vi "C8855-01_ReadData.vi"(8 "MainD":T1 {"G_DIM" format="%.5f"}) -> (0 "MainDR":T1 {"G_DIM" format="%.5f"}, 1 "RR2":u8, 2 "RR1":u8, 3 "Error":bool)   [LabVIEW 2017]
uses:
  C8855_MainD.ctl
  C8855-01api.dll
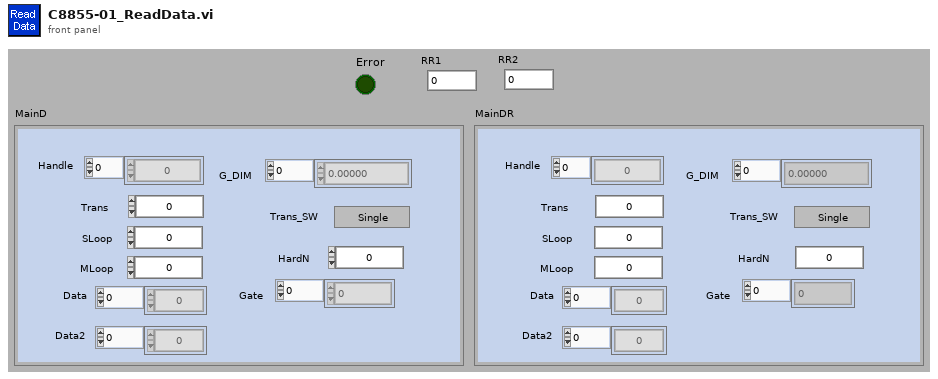
[diagram p1: front panel]
types:
  T1 = typedef "C8855_MainD.ctl" = cluster{"Handle":i64[], "G_DIM":dbl[], "Trans":u16, "Trans_SW":bool, "HardN":i32, "Gate":u8[], "Data":u32[], "Data2":u32[], "SLoop":i32, "MLoop":i32}
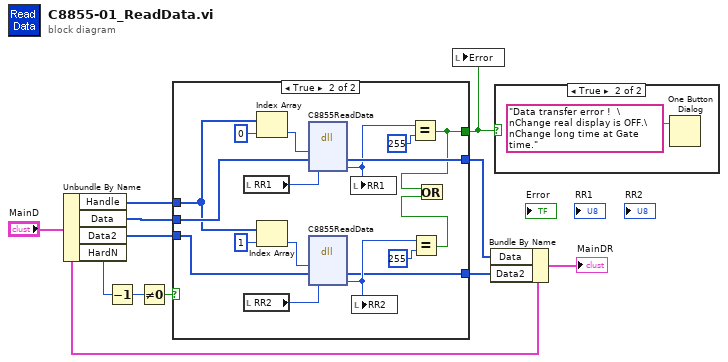
[diagram p0: block diagram]
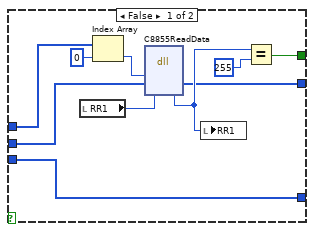
[diagram p3: hidden frame]
diagram:
  n1 = Unbundle By Name("MainD") -> ("Handle"=w9:i64[], "Data"=w7:u32[], "Data2"=w6:u32[], "HardN"=w8:i32)
  n2 = Decrement(x=w8) -> (x-1=w11:i32)
  n3 = Not Equal To 0?(x=w11) -> (x != 0?=w10:bool)
  n4 = case shown="True" w10 {
    tunnel: w9 -> [w21 w30]
    tunnel: w7 -> [w19 w37]
    tunnel: [w12 w34] -> w5
    tunnel: [w14 w23] -> w3
    tunnel: w6 -> [w13 w28]
    tunnel: [w13 w22] -> w4
    frame False {
      n5 = local read "RR1"() -> (w18:u8)
      n6 = Index Array(array=w21, index=0 ("Žw•W")) -> (element=w17:i64)
      n7 = dll-call lib="C:/Users/PC33412/Desktop/CD_Ver3.3.0/Sample/Source/x64/C8855-01api.dll" fn="C8855ReadData"("Handle"=w17, "Data Buffer"=w19, "ResultReturned"=w18) -> ("Data Buffer"=w12:u32[], "ResultReturned"=w15:u8)  [unwired: 4 in, 3 out]
      n8 = local write "RR1"(w15) -> ()
      n9 = Equal?(x=w15, y=u8 255) -> (x = y?=w14:bool)
    }
    frame True {
      n10 = local read "RR1"() -> (w36:u8)
      n11 = local read "RR2"() -> (w27:u8)
      n12 = Index Array(array=w30, index=0 ("Žw•W")) -> (element=w35:i64)
      n13 = Index Array(array=w30, index=1 ("Žw•W")) -> (element=w29:i64)
      n14 = dll-call lib="C:/Users/PC33412/Desktop/CD_Ver3.3.0/Sample/Source/x64/C8855-01api.dll" fn="C8855ReadData"("Handle"=w35, "Data Buffer"=w37, "ResultReturned"=w36) -> ("Data Buffer"=w34:u32[], "ResultReturned"=w32:u8)  [unwired: 4 in, 3 out]
      n15 = dll-call lib="C:/Users/PC33412/Desktop/CD_Ver3.3.0/Sample/Source/x64/C8855-01api.dll" fn="C8855ReadData"("Handle"=w29, "Data Buffer"=w28, "ResultReturned"=w27) -> ("Data Buffer"=w22:u32[], "ResultReturned"=w25:u8)  [unwired: 4 in, 3 out]
      n16 = local write "RR1"(w32) -> ()
      n17 = local write "RR2"(w25) -> ()
      n18 = Equal?(x=w32, y=u8 255) -> (x = y?=w23:bool)
      n19 = Equal?(x=w25, y=u8 255) -> (x = y?=w24:bool)
      n20 = Or(x=w23, y=w24) -> ()  [unwired: 1 out]
    }
  }
  n21 = local write "Error"(w3) -> ()
  n22 = Bundle By Name(cluster="MainD", "Data"=w5, "Data2"=w4) -> (→"MainDR":T1)
  n23 = case shown="True" w3 {
    frame False {
    }
    frame True {
      n24 = One Button Dialog(message="Data transfer error !  \nChange real display is OFF.\nChange long time at Gate time." ("爷景嫁")) -> ()  [unwired: 2 out]
    }
  }
